vi "SetGetReflector - Test.vi"() -> ()   [LabVIEW 2017]
uses:
  AT901 API/TypeDefinitions/ES_ReflectorType.ctl
panel:
  out "Command 2":string
  out "Respond 2":string[](array[string])
  in  "ES ReflectorType 2":T1=enum."CCR - 1,5 in"
  out "Command":string
  out "Respond":string[](array[string])
  out "ES ReflectorType":T1=enum."CCR - 1,5 in"
  out "error out":errorcluster
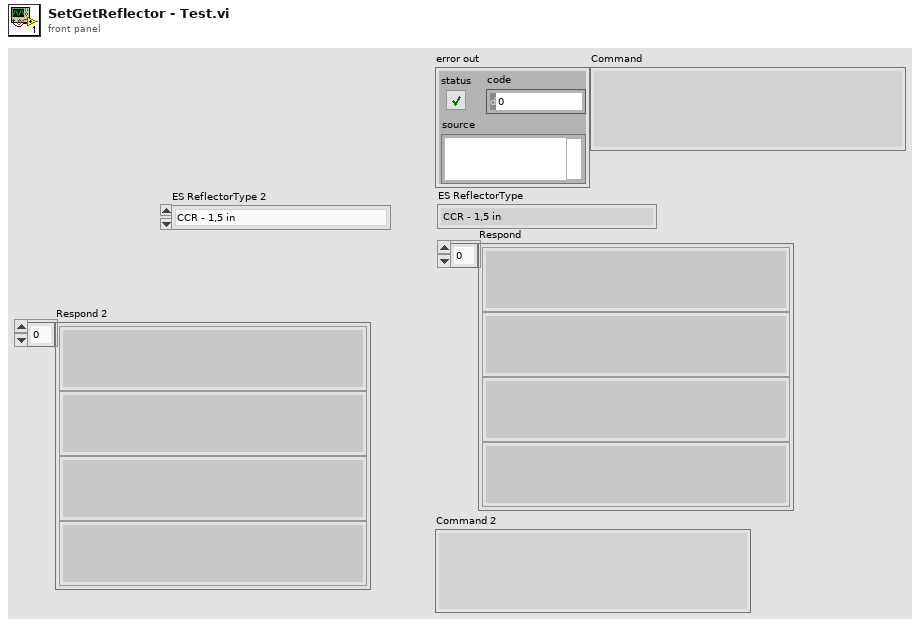
[diagram p1: front panel]
types:
  T1 = typedef "ES_ReflectorType.ctl" = enum32{"none1", "none2", "CCR - 1,5 in", "none4", "none5", "TBR - 0,5 in", "none7", "CCR - 75mm", "none8", "RRR - 1,5 in"}
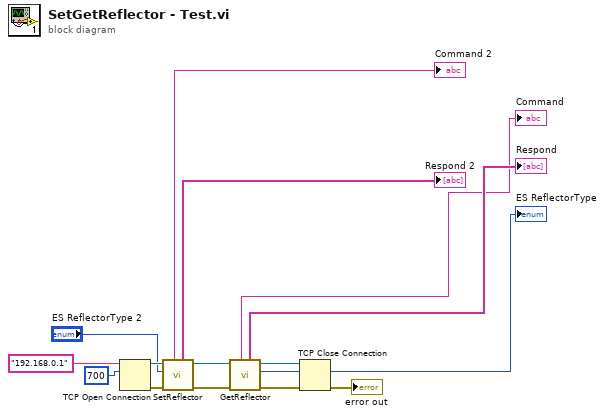
[diagram p0: block diagram]
diagram:
  n1 = TCP Open Connection(address="192.168.0.1", remote port or service name=u16 700) -> (connection ID=w12:refnum<k5>, error out=w7:errorcluster)  [unwired: 3 in]
  n2 = call "SetReflector.vi"("error in (no error)"=w7, "ES ReflectorType"="ES ReflectorType 2", "TCP Network Connection in"=w12) -> ("error out"=w8:errorcluster, "TCP Network Connection out"=w10:refnum<k5>, "Respond"=→"Respond 2":string[], "Command"=→"Command 2":string)  [unwired: 5 in]
  n3 = call "GetReflector.vi"("error in (no error)"=w8, "TCP Network Connection in"=w10) -> ("error out"=w9:errorcluster, "ES ReflectorType"=→"ES ReflectorType":T1, "TCP Network Connection out"=w11:refnum<k5>, "Respond"=→"Respond":string[], "Command"=→"Command":string)  [unwired: 5 in]
  n4 = TCP Close Connection(connection ID=w11, error in (no error)=w9) -> (error out=→"error out":errorcluster)  [unwired: 1 in, 1 out]
